vi "Test Controller.vi"(8 "error in":errorcluster) -> ()   [LabVIEW 2015]
doc: "This VI executes continuously carrying out the current operation and responding to updates or new operations. It will often contain the timing or control code that is difficult to place directly in TeleOp. This VI generally opens all sensors and motors and isolates the rest of the robot code from knowing how the operations are carried out."
uses:
  <vilib>/Rock Robotics/WPI/CAN/TalonSRX/WPI_CANTalonSRX_GlobalStatus.ctl
  Test Setpoints.ctl
  Test Operations.ctl
  <vilib>/Rock Robotics/WPI/CAN/TalonSRX/WPI_CANTalonSRX_APIControlMode.ctl
  <vilib>/Rock Robotics/WPI/CAN/TalonSRX/WPI_CANTalonSRX_APIFeedbackSelect.ctl
  <vilib>/Rock Robotics/WPI/MotorControl/WPI_MotorControlOpenCANTalonSRX.vi
  <vilib>/Rock Robotics/Network Tables/NT Write Boolean.vi
panel:
  out "Encoder RPS":dbl
  out "Talon SRX Status":T1 {"Encoder Position" format="%#_20g"}
  out "Current\nCmd":string
  # "Tip: It may be helpful to observe inputs and sensor values.\nYou may also want to display tuning or debugging controls."
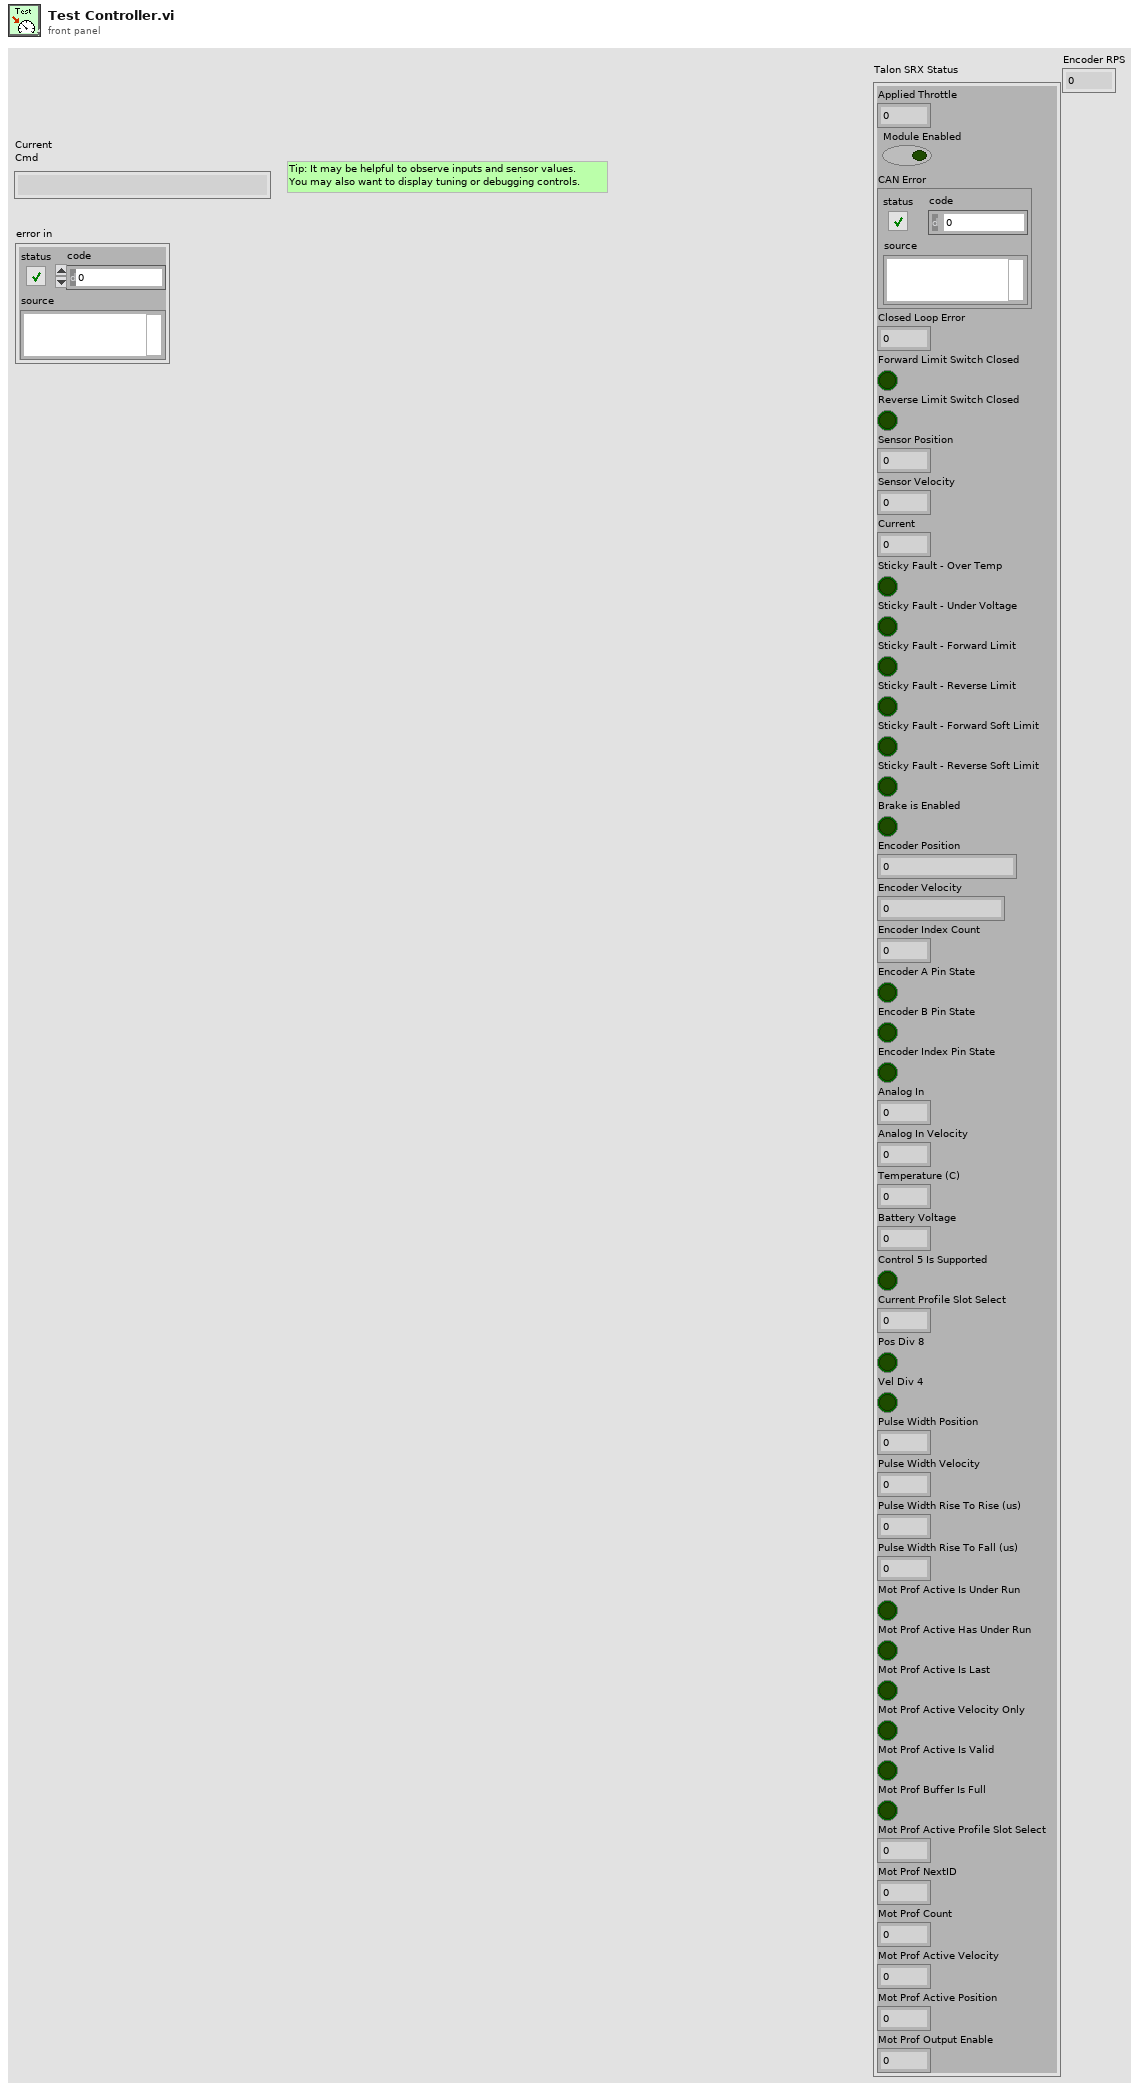
[diagram p1: front panel]
types:
  T1 = typedef "WPI_CANTalonSRX_GlobalStatus.ctl" = cluster{"Applied Throttle":dbl, "Module Enabled":bool, "CAN Error":errorcluster, "Closed Loop Error":dbl, "Forward Limit Switch Closed":bool, "Reverse Limit Switch Closed":bool, "Sensor Position":dbl, "Sensor Velocity":dbl, "Current":dbl, "Sticky Fault - Over Temp":bool, "Sticky Fault - Under Voltage":bool, "Sticky Fault - Forward Limit":bool, "Sticky Fault - Reverse Limit":bool, "Sticky Fault - Forward Soft Limit":bool, "Sticky Fault - Reverse Soft Limit":bool, "Brake is Enabled":bool, "Encoder Position":dbl, "Encoder Velocity":dbl, "Encoder Index Count":dbl, "Encoder A Pin State":bool, "Encoder B Pin State":bool, "Encoder Index Pin State":bool, "Analog In":dbl, "Analog In Velocity":dbl, "Temperature (C)":dbl, "Battery Voltage":dbl, "Control 5 Is Supported":bool, "Current Profile Slot Select":dbl, "Pos Div 8":bool, "Vel Div 4":bool, "Pulse Width Position":i32, "Pulse Width Velocity":i32, "Pulse Width Rise To Rise (us)":i32, "Pulse Width Rise To Fall (us)":i32, "Mot Prof Active Is Under Run":bool, "Mot Prof Active Has Under Run":bool, "Mot Prof Active Is Last":bool, "Mot Prof Active Velocity Only":bool, "Mot Prof Active Is Valid":bool, "Mot Prof Buffer Is Full":bool, "Mot Prof Active Profile Slot Select":i32, "Mot Prof NextID":i32, "Mot Prof Count":i32, "Mot Prof Active Velocity":dbl, "Mot Prof Active Position":dbl, "Mot Prof Output Enable":i32}
  T2 = typedef "WPI_CANTalonSRX_APIFeedbackSelect.ctl" = enum16{"Digital Quadrature Encoder", "Analog Potentiometer", "Analog Encoder", "Count on Quad-A (Rising-Edge)", "Count on Quad-A (Falling-Edge)", "CTR Magnetic Enc (Absolute)", "CTR Magnetic Enc (Relative)", "Pulse Width"}
  T3 = typedef "WPI_CANTalonSRX_APIControlMode.ctl" = enum8{"Percent VBus", "Speed", "Position", "Slave", "Unchanged / Invalid", "Voltage Compensation", "Current", "Motion Profile"}
  T4 = typedef "Test Setpoints.ctl" = cluster{"Operation":T5, "Setpoint":dbl, "Duration":dbl}
  T5 = typedef "Test Operations.ctl" = enum16{"Reserve", "Read Current", "Immediate", "Test PID Motor"}
  T6 = typedef "WPI_MotorControlDeviceRef.ctl" = cluster{"DeviceStatus":errorcluster, "Type":T7, "PWM":cluster{"PWM Channel":T8, "DeadBand":T9}, "CAN":cluster{"Device Number":u8, "Control Mode":T10, "Semaphore":T11, "Max Vout":dbl, "TalonSRX Control Mode":T3}, "Invert":bool}
  T7 = typedef "WPI_MotorControlType.ctl" = enum16{"PWM", "CAN", "CANTalonSRX"}
  T8 = typedef "FPGA_DIOPWMChannel.ctl" = enum8{"PWM 0", "PWM 1", "PWM 2", "PWM 3", "PWM 4", "PWM 5", "PWM 6", "PWM 7", "PWM 8", "PWM 9", "PWM MXP 0", "PWM MXP 1", "PWM MXP 2", "PWM MXP 3", "PWM MXP 4", "PWM MXP 5", "PWM MXP 6", "PWM MXP 7", "PWM MXP 8", "PWM MXP 9", "Invalid"}
  T9 = typedef "WPI_PWMDeadband.ctl" = cluster{"Name":string, "maxPositivePwm":i32, "minPositivePwm":i32, "centerPwm":i32, "maxNegativePwm":i32, "minNegativePwm":i32, "angularRange":u16}
  T10 = typedef "WPI_CANJaguar_ControlMode.ctl" = enum8{"Percent VBus", "Current", "Speed", "Position", "Voltage"}
  T11 = typedef "Semaphore RefNum" = refnum<k1>
  T12 = typedef "Command Status Info.ctl" = cluster{"Name":string, "Status":T13, "notifier out":T14}
  T13 = typedef "Completion Status.ctl" = enum16{"Successful", "Aborted", "Incomplete"}
  T14 = typedef "Completion Notifier.ctl" = refnum<notifier>
  T15 = cluster{"Default Command":T4, "Command Timing":cluster{"Start Time (ms)":u32, "Iterations":i32}, "Command Arguments":cluster{"Command Info":T12, "Description":string, "Default Command":T4, "notifier out":refnum<notifier>, "Subsystem Name":string}}
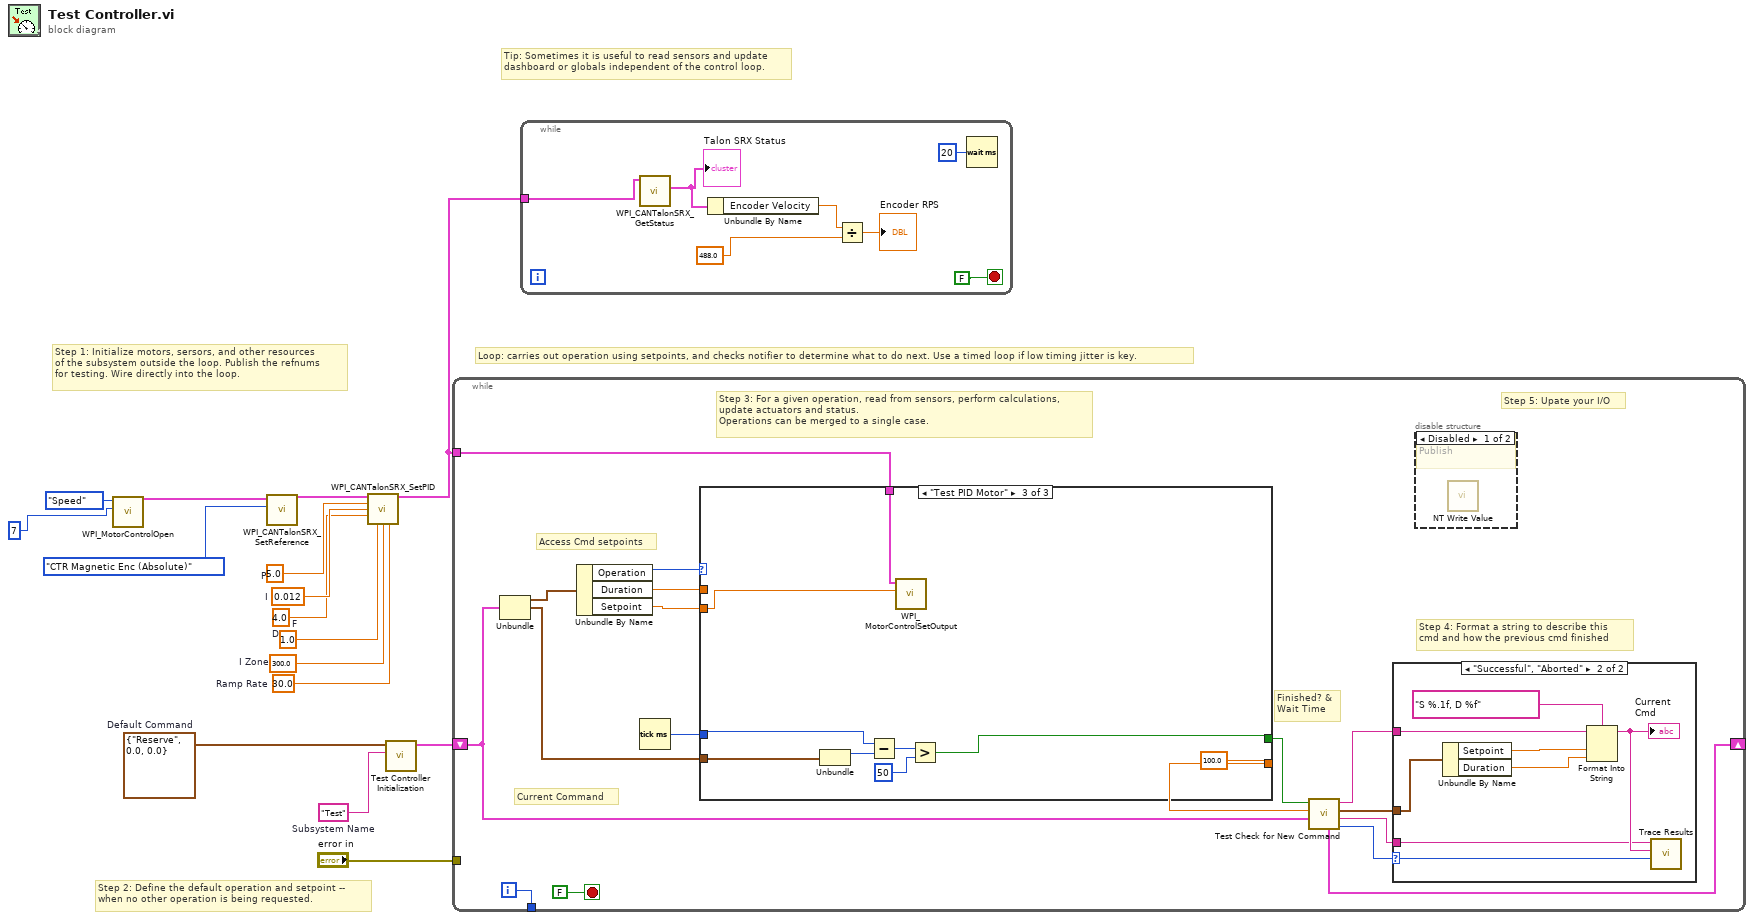
[diagram p0: block diagram]
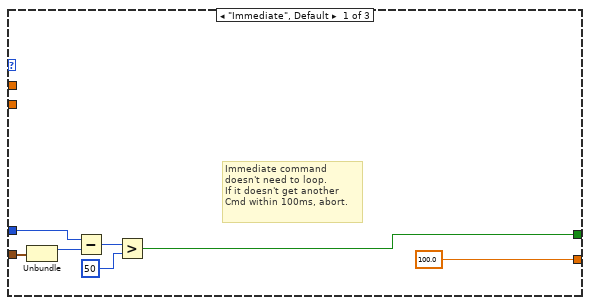
[diagram p4: hidden frame]
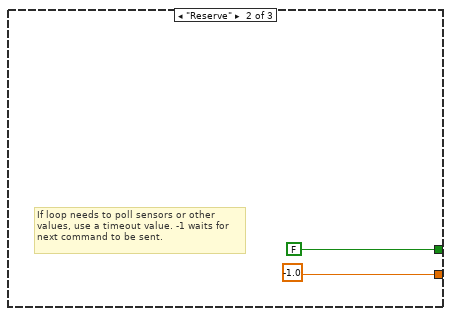
[diagram p5: hidden frame]
diagram:
  w2 = 30.0  # Ramp Rate
  w3 = 300.0  # I Zone
  w4 = 1.0  # F
  w5 = 4.0  # D
  w6 = 0.012  # I
  w7 = 5.0  # P
  w13 = T4 {"Operation"=enum."Reserve", "Setpoint"=0.0, "Duration"=0.0}  # Default Command
  w14 = "Test"  # Subsystem Name
  # "Tip: Sometimes it is useful to read sensors and update\ndashboard or globals independent of the control loop."
  # "Step 2: Define the default operation and setpoint --\nwhen no other operation is being requested."
  # "Step 1: Initialize motors, sersors, and other resources\nof the subsystem outside the loop. Publish the refnums\nfor testing. Wire directly into the loop."
  # "Loop: carries out operation using setpoints, and checks notifier to determine what to do next. Use a timed loop if low timing jitter is key."
  n1 = call-poly <vilib>:"WPI_MotorControlOpen.vi"("Device Number"=u8 7, "Control Mode"=WPI_CANTalonSRX_APIControlMode."Speed") -> ("MotorControlDeviceRef"=w9:T6)  [unwired: 8 in, 1 out]
  n2 = call <vilib>:"WPI_CANTalonSRX_SetReference.vi"("Feedback Reference"=WPI_CANTalonSRX_APIFeedbackSelect."CTR Magnetic Enc (Absolute)", "CAN Talon SRX Ref"=w9) -> ("CAN Talon SRX Ref"=w8:T6)  [unwired: 8 in, 1 out]
  n3 = call <vilib>:"WPI_CANTalonSRX_SetPID.vi"("CAN Talon SRX Ref"=w8, "P"=w7, "I"=w6, "D"=w5, "F"=w4, "I Zone"=w3, "Ramp Rate"=w2) -> ("CAN Talon SRX Ref"=w1:T6)  [unwired: 7 in, 1 out]
  n4 = call "Test Controller Initialization.vi"("Subsystem Name"=w14, "Default Command"=w13) -> ("Command Info"=w15:T15)  [unwired: 9 in]
  n5 = while {
    shift-right: [w24] -> _
    shift-left: w15 -> [w25]
    tunnel: [w32] -> _
    tunnel: "error in" -> [_]
    tunnel: w1 -> [w17]
    i -> [w32]
    stop <- FALSE stop-if-true
    # "Step 5: Upate your I/O"
    # "Step 4: Format a string to describe this\ncmd and how the previous cmd finished"
    # "Current Command"
    # "Access Cmd setpoints"
    # "Finished? &\nWait Time"
    # "Step 3: For a given operation, read from sensors, perform calculations,\nupdate actuators and status.\nOperations can be merged to a single case."
    n6 = Unbundle(w25) -> ("Default Command"=w31:T4, "Command Timing"=w27:cluster{"Start Time (ms)":u32, "Iterations":i32})  [unwired: 1 out]
    n7 = Unbundle By Name(w31) -> ("Operation"=w30:T5, "Duration"=w29:dbl, "Setpoint"=w26:dbl)
    n8 = Tick Count (ms)() -> (millisecond timer value=w28:u32)
    n9 = case shown="\"Test PID Motor\"" w30 {
      tunnel: [100.0 -1.0 100.0] -> w22
      tunnel: [w42 FALSE ("ignore previous (F)") w51] -> w23
      tunnel: w27 -> [w44 _ w53]
      tunnel: w29 -> [_ _ _]
      tunnel: w28 -> [w43 _ w54]
      tunnel: w26 -> [_ _ w58]
      tunnel: w17 -> [_ _ w59]
      frame "Immediate", Default {
        # "Immediate command\ndoesn't need to loop.\nIf it doesn't get another\nCmd within 100ms, abort."
        n10 = Unbundle(w44) -> ("Start Time (ms)"=w47:u32)  [unwired: 1 out]
        n11 = Subtract(x=w43, y=w47) -> (x-y=w46:u32)
        n12 = Greater?(x=w46, y=u8 50 ("Left Motor")) -> (0:w42:bool)
      }
      frame "Reserve" {
        # "If loop needs to poll sensors or other\nvalues, use a timeout value. -1 waits for\nnext command to be sent."
      }
      frame "Test PID Motor" {
        n13 = Unbundle(w53) -> ("Start Time (ms)"=w57:u32)  [unwired: 1 out]
        n14 = Subtract(x=w54, y=w57) -> (x-y=w56:u32)
        n15 = call <vilib>:"WPI_MotorControlSetOutput.vi"("Output"=w58, "MotorControlDevRef"=w59) -> ()  [unwired: 7 in, 3 out]
        n16 = Greater?(x=w56, y=u8 50 ("Left Motor")) -> (0:w51:bool)
      }
    }
    n17 = call "Test Check for New Command.vi"("Current Command"=w25, "Wait time (ms)"=w22, "Finished?"=w23) -> ("Completion"=w18:T13, "Subsystem Name"=w19:string, "Current Command"=w20:T4, "Initial Trace String"=w21:string, "NextCommand"=w24:T15)  [unwired: 4 in]
    n18 = case shown="\"Successful\", \"Aborted\"" w18 {
      selector: w18 -> [_ w41]
      tunnel: w21 -> [_ w37]
      tunnel: w20 -> [_ w38]
      tunnel: w19 -> [_ w34]
      frame "Incomplete", Default {
        # "Continuing current command"
      }
      frame "Successful", "Aborted" {
        # "Report and setup for next command"
        n19 = Unbundle By Name(w38) -> ("Setpoint"=w40:dbl, "Duration"=w35:dbl)
        n20 = Format Into String(format string="S %.1f, D %f", initial string=w37, w40, w35) -> (resulting string=w36:string)  [unwired: 1 in, 1 out]
        "Current\nCmd" <- w36
        n21 = call <vilib>:"Trace Results.vi"("Status of previous command"=w41, "Description"=w36, "Subsystem"=w34) -> ()  [unwired: 9 in]
      }
    }
    n22 = disable-structure shown="Disabled" {
      frame Disabled {
        # "Publish"
        n23 = call-poly <vilib>:"NT Write Value.vi"() -> ()  [unwired: 11 in, 1 out]
      }
      frame Enabled {
      }
    }
  }
  n24 = while {
    tunnel: w1 -> [w64]
    stop <- FALSE stop-if-true
    n25 = call <vilib>:"WPI_CANTalonSRX_GetStatus.vi"("CAN Talon SRX Ref"=w64) -> ("Talon SRX Status"=w63:T1)  [unwired: 8 in, 2 out]
    "Talon SRX Status" <- w63
    n26 = Unbundle By Name(w63) -> ("Encoder Velocity"=w61:dbl)
    n27 = Divide(x=w61, y=488.0) -> (x/y=→"Encoder RPS":dbl)
    n28 = Wait (ms)(milliseconds to wait=u32 20) -> ()  [unwired: 1 out]
  }
